vi "Measure in Background.vi"(5 "Buffer 1":string, 6 "Buffer 2":string, 7 "Function (Current)":T1(ring), 8 "error in (no error)":errorcluster, 9 "Channel (Channel A)":T2, 10 "Node In":string, 11 "VISA resource name":refnum<visa-resource-name>) -> (0 "error out":errorcluster, 2 "Node Out":string, 3 "VISA resource name out":refnum<visa-resource-name>, 4 "Command String":string)   [LabVIEW 2009, in "Keithley 2600 Series.lvlib"]
doc: "This VI starts an asynchronous (background) measurement.\n\nThis function will start a measurement and return immediately. The measurements, as they are performed, are stored in a reading buffer (along with any ancillary information also being acquired). If the instrument is configured to return multiple readings where one is requested, the readings will be available as they are made.\n\n<b>Note:</b> Reading buffers are required for overlapped measurements.\n\n<b>Functions and Attributes Used</b>\nsmuX.measure.overlappedY(rbuffer)\nsmuX.measure.overlappediv(ibuffer, vbuffer)"
uses:
  <instrlib>/Keithley 2600 Series/Keithley 2600 Series.lvlib
  <instrlib>/Keithley 2600 Series/Public/Channel.ctl
  <instrlib>/Keithley 2600 Series/Private/GlobalVariables.vi
panel:
  # "(c) 2008 Keithley Instruments, Inc.  ALL RIGHTS RESERVED."
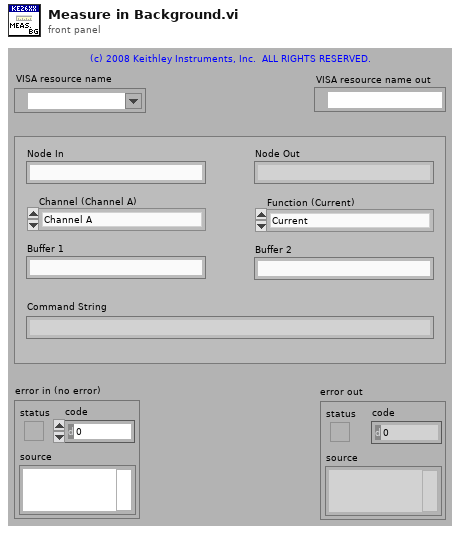
[diagram p1: front panel]
types:
  T1 = enum32{"Current", "Voltage", "IV", "Resistance", "Power"}
  T2 = typedef "Keithley 2600 Series.lvlib/Channel.ctl" = enum32{"Channel A", "Channel B"}
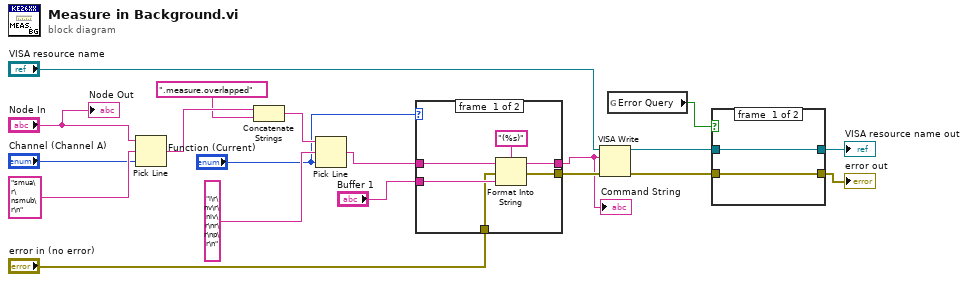
[diagram p0: block diagram]
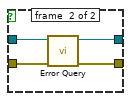
[diagram p2: hidden frame]
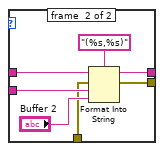
[diagram p3: hidden frame]
diagram:
  n1 = Pick Line(string ("")="Node In", multi-line string="smua\r\nsmub\r\n" ("options"), line index="Channel (Channel A)") -> (output string=w17:string)
  n2 = Concatenate Strings(w17, ".measure.overlapped" ("command")) -> (w15:string)
  n3 = Pick Line(string ("")=w15, multi-line string="i\r\nv\r\niv\r\nr\r\np\r\n" ("options"), line index="Function (Current)") -> (output string=w11:string)
  n4 = case shown="\"IV\"" "Function (Current)" {
    tunnel: w11 -> [w24 w31]
    tunnel: "Buffer 1" -> [w23 w30]
    tunnel: "error in (no error)" -> [w22 w28]
    tunnel: [w20 w27] -> w8
    tunnel: [w21 w26] -> w1
    frame #0 {
      n5 = Format Into String(format string="(%s)", initial string=w24, error in=w22, w23) -> (resulting string=w21:string, error out=w20:errorcluster)
    }
    frame #1 {
      n6 = Format Into String(format string="(%s,%s)", initial string=w31, error in=w28, w30, "Buffer 2") -> (resulting string=w26:string, error out=w27:errorcluster)
    }
  }
  "Command String" <- w1
  n7 = VISA Write(VISA resource name="VISA resource name", write buffer=w1, error in (no error)=w8) -> (VISA resource name out=w5:refnum<visa-resource-name>, error out=w4:errorcluster)  [unwired: 1 out]
  n8 = global read "GlobalVariables.vi" "Error Query"() -> (w6:bool)
  n9 = case shown="True" w6 {
    tunnel: w5 -> [w34 w38]
    tunnel: w4 -> [w33 w37]
    tunnel: [w34 w36] -> w3
    tunnel: [w33 w35] -> w2
    frame #0 {
    }
    frame #1 {
      n10 = call <instrlib>:"Error Query.vi"("error in (no error)"=w37, "VISA resource name"=w38) -> ("error out"=w35:errorcluster, "VISA resource name out"=w36:refnum<visa-resource-name>)  [unwired: 8 out]
    }
  }
  "VISA resource name out" <- w3
  "error out" <- w2
  "Node Out" <- "Node In"
